vi "update event data.vi"(8 "error in":errorcluster, 9 "varient in":variant, 10 "Command":string, 11 "refnum in":T1) -> (0 "error out":errorcluster, 3 "refnum in":T1)   [LabVIEW 2020, in "Publisher Subscriber.lvlib"]
uses:
  Publisher Subscriber.lvlib
  Controls/node refnum.ctl
  Controls/node dvr data.ctl
  Controls/data cluster.ctl
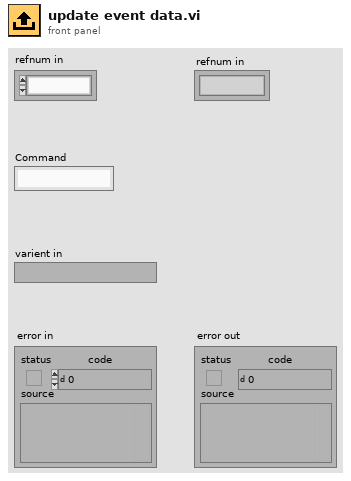
[diagram p1: front panel]
types:
  T1 = typedef "Publisher Subscriber.lvlib/node refnum.ctl" = refnum<k1>
  T2 = typedef "Publisher Subscriber.lvlib/node dvr data.ctl" = cluster{"queue ref":refnum<queue>, "subscription map ref":refnum<data-value>, "Command":string, "Data":variant, "Subscriptions []":set{string}, "variable dvr refs":refnum<data-value>}
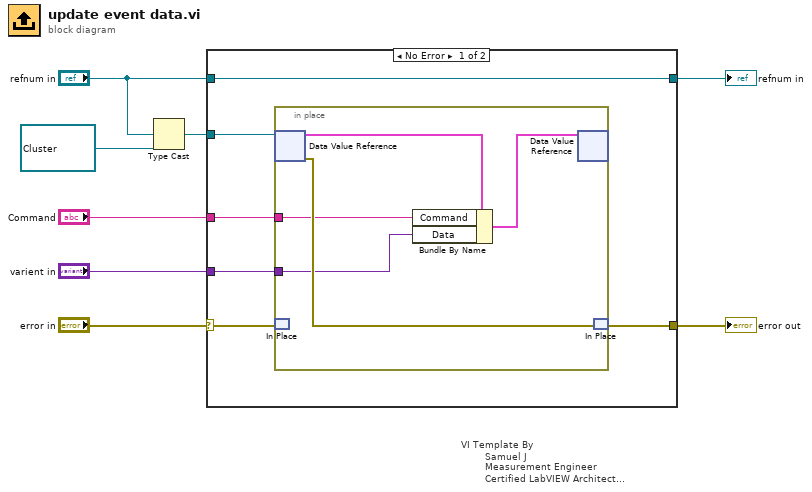
[diagram p0: block diagram]
diagram:
  n1 = Type Cast(type=refnum<data-value> refnum ("data value reference"), x="refnum in") -> (*(type *) &x=w5:refnum<data-value>)
  n2 = case "VI Template By\n        Samuel J\n        Measurement Engineer\n        Certified LabVIEW Architect\n        Vestas Technology R&D Chennai" shown="No Error" "error in" {
    selector: "error in" -> [w12 w21]
    tunnel: [w10 w21] -> w7
    tunnel: w5 -> [w13 _]
    tunnel: [w14 w20] -> w4
    tunnel: "refnum in" -> [w14 w20]
    tunnel: "varient in" -> [w11 _]
    tunnel: "Command" -> [w9 _]
    frame No Error {
      n3 = in-place {
        in-place-border: w11 -> [w17]
        in-place-border: w9 -> [w16]
        n4 = in-place-dvr #1(w13) -> (w18:T2, w19:errorcluster)
        n5 = in-place-match #2(w12) -> ()  [unwired: 1 out]
        n6 = Bundle By Name(cluster=w18, "Command"=w16, "Data"=w17) -> (w15:T2)
        n7 = in-place-dvr #1(w15) -> ()  [unwired: 2 out]
        n8 = in-place-match #2(w19) -> (w10:errorcluster)
      }
    }
    frame Error {
    }
  }
  "error out" <- w7
  "refnum in" <- w4
